vi "JSR SetReveive.vi"(8 "error in (no error)":errorcluster, 10 "JSR Receive Settings":T1={"Receiver Mode"=0, "High Pass Filter"=5000, "Low Pass Filter"=50, "Gain (dB)"=50} {"Gain (dB)" min=-13 max=66 step=1; "Low Pass Filter" items=["5 MHz"=5, "10 MHz"=10, "15 MHz"=15, "22.5 MHz"=22, "35 MHz"=35, "50 MHz"=50]; "High Pass Filter" items=["DC"=0, "1 MHz"=1000, "2.5 MHz"=2500, "5 MHz"=5000, "7.5 MHz"=7500, "12.5 MHz"=12500]; "Receiver Mode" items=["Echo", "Through"]}, 11 "VISA Refnum in":refnum<visa-resource-name>) -> (0 "error out":errorcluster, 3 "VISA Refnum out":refnum<visa-resource-name>)   [LabVIEW 2022 SP3]
uses:
  Controls/JSR Recieve.ctl
  Controls/Mode.ctl
  Controls/HPF.ctl
  Controls/LPF.ctl
  Controls/Gain.ctl
  PulserGlobals.vi
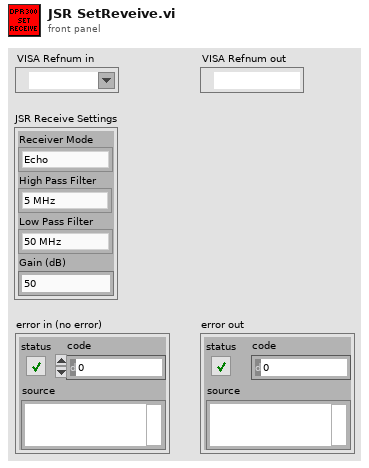
[diagram p1: front panel]
types:
  T1 = typedef "JSR Recieve.ctl" = cluster{"Receiver Mode":T2, "High Pass Filter":T3, "Low Pass Filter":T4, "Gain (dB)":T5}
  T2 = typedef "Mode.ctl" = i8
  T3 = typedef "HPF.ctl" = u16
  T4 = typedef "LPF.ctl" = u16
  T5 = typedef "Gain.ctl" = i8
  T6 = cluster{"Energy (microJ)":u8, "Damping (In Ohm)":u8, "HP Filt(KHz) ":u16, "LP Filt (MHz)":u8, "Gain (db)":u8, "Atten (dB)":sgl}
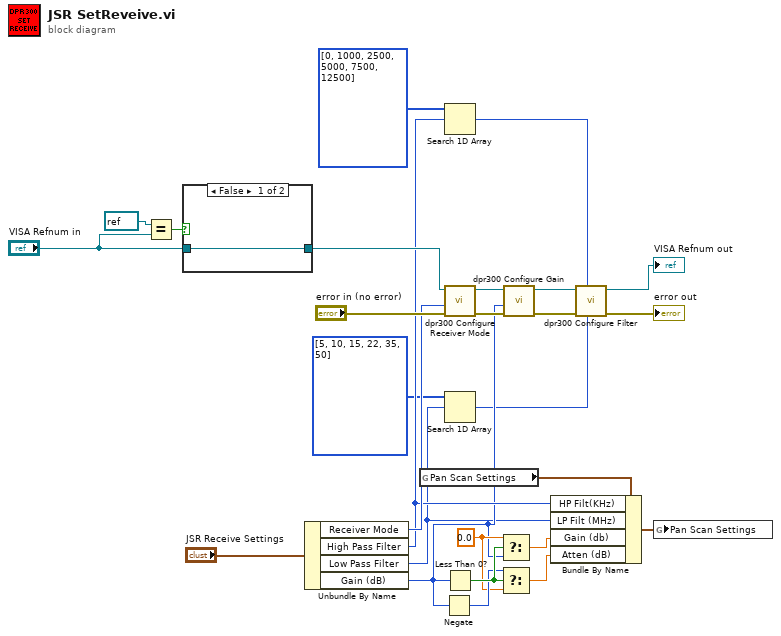
[diagram p0: block diagram]
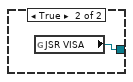
[diagram p2: hidden frame]
diagram:
  w3 = T4[] [5, 10, 15, 22, 35, 50] items=["5 MHz"=5, "10 MHz"=10, "15 MHz"=15, "22.5 MHz"=22, "35 MHz"=35, "50 MHz"=50]
  w7 = T3[] [0, 1000, 2500, 5000, 7500, 12500] items=["DC"=0, "1 MHz"=1000, "2.5 MHz"=2500, "5 MHz"=5000, "7.5 MHz"=7500, "12.5 MHz"=12500]
  w8 = 0.0 ("t")
  n1 = Equal?(x=refnum<visa-resource-name> refnum, y="VISA Refnum in") -> (x = y?=w17:bool)
  n2 = case shown="False" w17 {
    tunnel: [w28 w29] -> w16
    tunnel: "VISA Refnum in" -> [w28 _]
    frame False {
    }
    frame True {
      n3 = global read "PulserGlobals.vi" "JSR VISA"() -> (w29:refnum<visa-resource-name>)
    }
  }
  n4 = Unbundle By Name("JSR Receive Settings") -> ("Receiver Mode"=w24:T2, "High Pass Filter"=w6:T3, "Low Pass Filter"=w2:T4, "Gain (dB)"=w5:T5)
  n5 = global read "PulserGlobals.vi" "Pan Scan Settings"() -> (w14:T6)
  n6 = Negate(x=w5) -> (-x=w10:T5)
  n7 = Search 1D Array(1D array=w7, element=w6) -> (index of element=w4:i32)  [unwired: 1 in]
  n8 = call <instrlib>:"dpr300 Configure Receiver Mode.vi"("error in (no error)"="error in (no error)", "Receiver Mode (0: Echo)"=w24, "VISA resource name"=w16) -> ("error out"=w20:errorcluster, "VISA resource name out"=w19:refnum<visa-resource-name>)  [unwired: 7 in]
  n9 = Search 1D Array(1D array=w3, element=w2) -> (index of element=w1:i32)  [unwired: 1 in]
  n10 = Less Than 0?(x=w5) -> (x < 0?=w12:bool)
  n11 = Select(t=w8, s=w12, f=w5) -> (s? t:f=w11:dbl)
  n12 = Select(t=w10, s=w12, f=w8) -> (s? t:f=w9:dbl)
  n13 = call <instrlib>:"dpr300 Configure Gain.vi"("error in (no error)"=w20, "Gain (50 dB)"=w5, "VISA resource name"=w19) -> ("error out"=w27:errorcluster, "VISA resource name out"=w26:refnum<visa-resource-name>)  [unwired: 7 in]
  n14 = Bundle By Name(cluster=w14, "HP Filt(KHz)"=w6, "LP Filt (MHz)"=w2, "Gain (db)"=w11, "Atten (dB)"=w9) -> (w13:T6)
  n15 = call <instrlib>:"dpr300 Configure Filter.vi"("Low Pass Filter (3: 15 / 22.5 MHz)"=w1, "High Pass Filter (3: 5 MHz)"=w4, "error in (no error)"=w27, "VISA resource name"=w26) -> ("error out"=→"error out":errorcluster, "VISA resource name out"=→"VISA Refnum out":refnum<visa-resource-name>)  [unwired: 6 in]
  n16 = global write "PulserGlobals.vi" "Pan Scan Settings"(w13) -> ()
